vi "Flatten Value.vi"(8 "Error In":errorcluster, 11 "String In":refnum<class "String.lvclass">) -> (0 "Error Out":errorcluster, 1 "Value":string, 3 "String Out":refnum<class "String.lvclass">)   [LabVIEW 2017, in "Tree API.lvlib" / "String.lvclass"]
uses:
  String.lvclass
  Tree Manager/Tree.lvclass
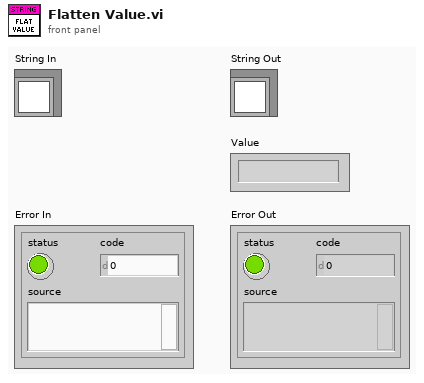
[diagram p1: front panel]
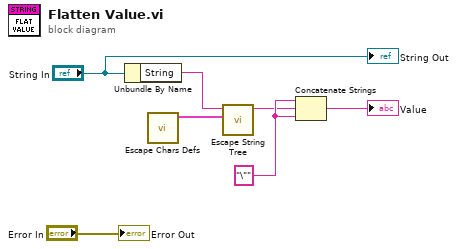
[diagram p0: block diagram]
diagram:
  w5 = "\"" ("string")
  n1 = Unbundle By Name("String In") -> ("String"=w3:string)
  n2 = call "Escape Chars Defs.vi"() -> ("Escapes"=w4:cluster{"String":string, "Escape":string}[])  [unwired: 11 in]
  n3 = call "Escape String Tree.vi"("Escapes"=w4, "String In"=w3) -> ("String Out"=w2:string)  [unwired: 9 in]
  n4 = Concatenate Strings(w5, w2, w5) -> (→"Value":string)
  "String Out" <- "String In"
  "Error Out" <- "Error In"
